vi "RXMux-Direct.vi"() -> ()   [LabVIEW 2009]
uses:
  <vilib>/NXT/Subs/LVHSConnector.ctl
  <vilib>/NXT/Block Support/NXT_InputPort.ctl
panel:
  in  "Channe to  Select":u8(ring) items=["Read Channel", "Select Ch1", "Select Ch2", "Select Ch3", "Select Ch4"]
  out "NXT dup":T1
  in  "Input Port":T2 items=["Port 1", "Port 2", "Port 3", "Port 4"]
  out "Light":i16=14 caption="Scaled Value"
  in  "stop":bool
  in  "NXT":T1
  # "mindsensors.com\nCopyright (c) 2009 by mindsensors.com\nEmail: info (<at>) mindsensors (<dot>) com\n\nThis program is free software. You can redistribute it and/or modify\nit under the terms of the GNU General Public License as published by\nthe Free Software Foundation; version 3 of the License.\nRead the license at: http://www.gnu.org/licenses/gpl.txt"
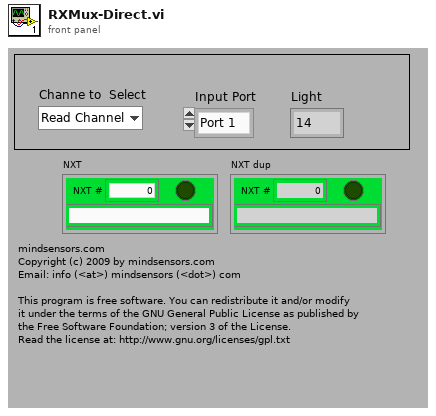
[diagram p1: front panel]
types:
  T1 = typedef "LVHSConnector.ctl" = cluster{"error":errorcluster, "address":string, "NXT #":i32, "Show Error":bool}
  T2 = typedef "NXT_InputPort.ctl" = u8
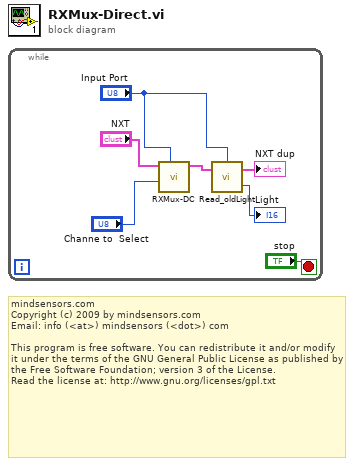
[diagram p0: block diagram]
diagram:
  # "mindsensors.com\nCopyright (c) 2009 by mindsensors.com\nEmail: info (<at>) mindsensors (<dot>) com\n\nThis program is free software. You can redistribute it and/or modify\nit under the terms of the GNU General Public License as published by\nthe Free Software Foundation; version 3 of the License.\nRead the license at: http://www.gnu.org/licenses/gpl.txt"
  n1 = while {
    stop <- "stop" stop-if-true
    n2 = call "RXMux-DC.vi"("Input Port"="Input Port", "Channe to  Select"="Channe to  Select", "NXT"="NXT") -> ("NXT dup"=w6:T1)  [unwired: 7 in, 1 out]
    n3 = call <vilib>:"Read_oldLight.vi"("NXT"=w6, "Port (Port 3)"="Input Port") -> ("light"=→"Light":i16, "NXT"=→"NXT dup":T1)  [unwired: 1 in]
  }
